vi "未命名 4.vi"   [LabVIEW 2018]
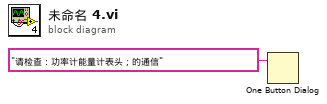
[diagram p0: block diagram]
diagram:
  n1 = One Button Dialog(message="请检查：功率计能量计表头；的通信" ("消息")) -> ()  [unwired: 1 in, 1 out]
